vi "Canwrite_jetson_R.vi"(10 "Control param in":T1) -> (2 "배열":T2(array[cluster]))   [LabVIEW 2019]
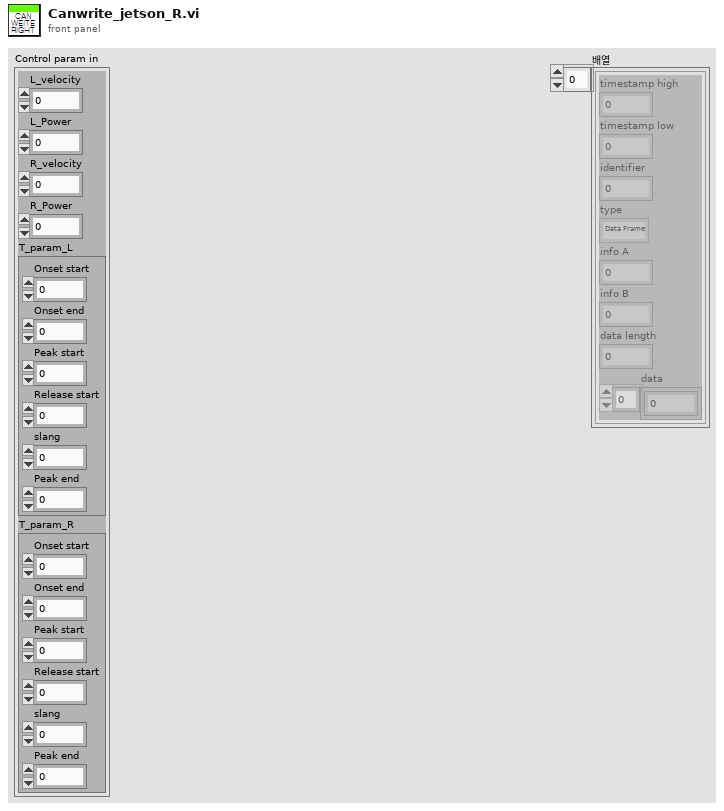
[diagram p1: front panel]
types:
  T1 = cluster{"L_velocity":u32, "L_Power":sgl, "R_velocity":u32, "R_Power":sgl, "T_param_L":cluster{"Onset start":sgl, "Onset end":sgl, "Peak start":sgl, "Release start":sgl, "slang":sgl, "Peak end":sgl}, "T_param_R":cluster{"Onset start":sgl, "Onset end":sgl, "Peak start":sgl, "Release start":sgl, "slang":sgl, "Peak end":sgl}}
  T2 = cluster{"timestamp high":u32, "timestamp low":u32, "identifier":u32, "type":enum8{"Data Frame", "Remote Frame", "(reserved)", "(reserved) ", "(reserved)  ", "(reserved)   ", "Bus Error", "Transceiver Fault"}, "info A":u8, "info B":u8, "data length":u8, "data":u8[]}[]
  T3 = enum8{"Data Frame", "Remote Frame", "(reserved)", "(reserved) ", "(reserved)  ", "(reserved)   ", "Bus Error", "Transceiver Fault"}
  T4 = cluster{"timestamp high":u32, "timestamp low":u32, "identifier":u32, "type":enum8{"Data Frame", "Remote Frame", "(reserved)", "(reserved) ", "(reserved)  ", "(reserved)   ", "Bus Error", "Transceiver Fault"}, "info A":u8, "info B":u8, "data length":u8, "data":u8[]}
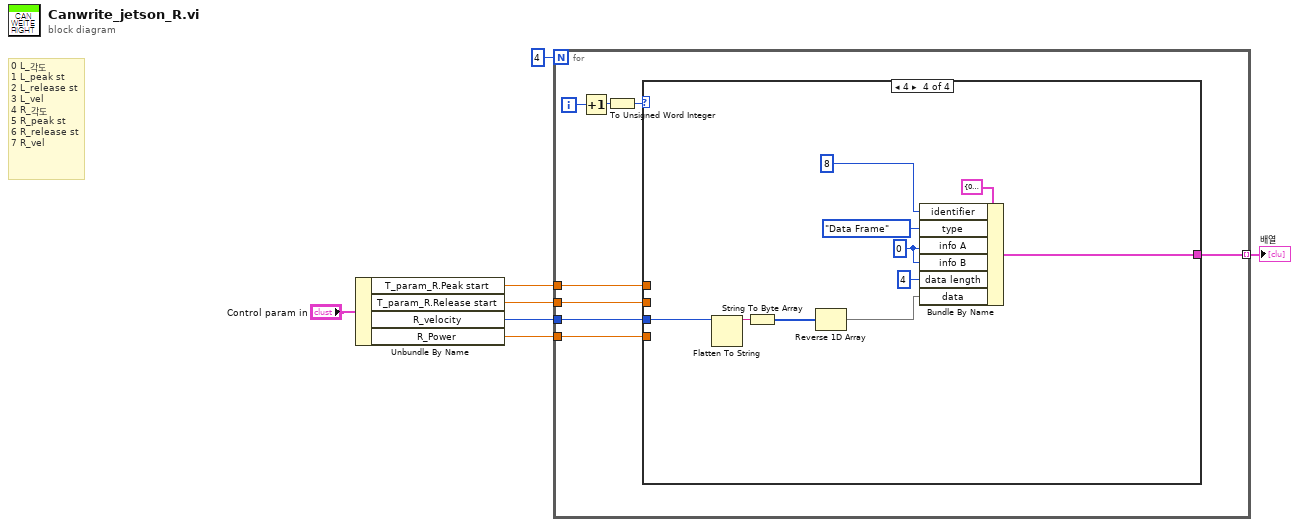
[diagram p0: block diagram]
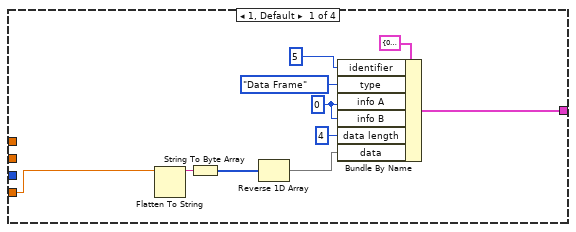
[diagram p2: hidden frame]
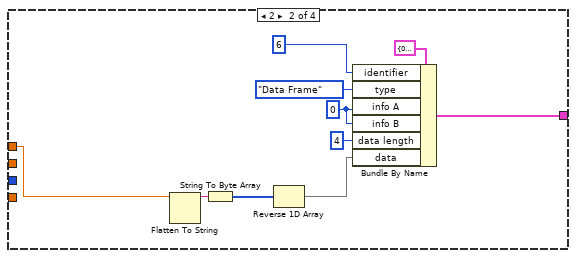
[diagram p3: hidden frame]
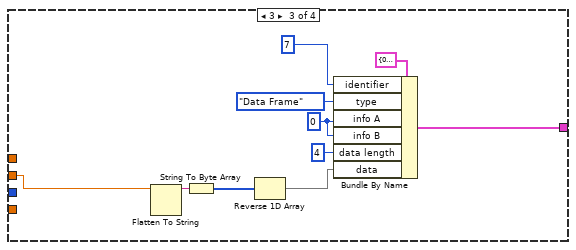
[diagram p4: hidden frame]
diagram:
  # "0 L_각도\n1 L_peak st\n2 L_release st\n3 L_vel\n4 R_각도\n5 R_peak st\n6 R_release st\n7 R_vel"
  n1 = Unbundle By Name("Control param in") -> ("T_param_R.Peak start"=w4:sgl, "T_param_R.Release start"=w3:sgl, "R_velocity"=w2:u32, "R_Power"=w1:sgl)
  n2 = for {
    N: 4 -> [_]
    tunnel: [w15] -> w6 mode=indexing
    tunnel: w4 -> [w11]
    tunnel: w3 -> [w10]
    tunnel: w2 -> [w9]
    tunnel: w1 -> [w8]
    i -> [w14]
    n3 = Increment(x=w14) -> (x+1=w13:i32)
    n4 = To Unsigned Word Integer(number=w13) -> (unsigned 16bit integer=w12:u16)
    n5 = case shown="4" w12 {
      tunnel: [w21 w31 w41 w51] -> w15
      tunnel: w11 -> [_ w27 _ _]
      tunnel: w10 -> [_ _ w37 _]
      tunnel: w9 -> [_ _ _ w47]
      tunnel: w8 -> [w17 _ _ _]
      frame 1, Default {
        w23 = u8 0 ("info A")
        n6 = Flatten To String(anything=w17) -> (data string=w20:string)  [unwired: 3 in, 2 out]
        n7 = String To Byte Array(string=w20) -> (unsigned byte array=w19:u8[])
        n8 = Reverse 1D Array(array=w19) -> (reversed array=w18:u8[])
        n9 = Bundle By Name(cluster=T4 {"timestamp high"=0, "timestamp low"=0, "identifier"=0, "type"=enum."Data Frame", "info A"=0, "info B"=0, "data length"=0, "data"=[0, 0, 0, 0, 0, 0, 0, 0]} ("출력 클러스터"), "identifier"=u32 5, "type"=T3."Data Frame", "info A"=w23, "info B"=w23, "data length"=u8 4, "data"=w18) -> (w21:T4)
      }
      frame 2 {
        w33 = u8 0 ("info A")
        n10 = Flatten To String(anything=w27) -> (data string=w30:string)  [unwired: 3 in, 2 out]
        n11 = String To Byte Array(string=w30) -> (unsigned byte array=w29:u8[])
        n12 = Reverse 1D Array(array=w29) -> (reversed array=w28:u8[])
        n13 = Bundle By Name(cluster=T4 {"timestamp high"=0, "timestamp low"=0, "identifier"=0, "type"=enum."Data Frame", "info A"=0, "info B"=0, "data length"=0, "data"=[0, 0, 0, 0, 0, 0, 0, 0]} ("출력 클러스터"), "identifier"=u32 6, "type"=T3."Data Frame", "info A"=w33, "info B"=w33, "data length"=u8 4, "data"=w28) -> (w31:T4)
      }
      frame 3 {
        w43 = u8 0 ("info A")
        n14 = Flatten To String(anything=w37) -> (data string=w40:string)  [unwired: 3 in, 2 out]
        n15 = String To Byte Array(string=w40) -> (unsigned byte array=w39:u8[])
        n16 = Reverse 1D Array(array=w39) -> (reversed array=w38:u8[])
        n17 = Bundle By Name(cluster=T4 {"timestamp high"=0, "timestamp low"=0, "identifier"=0, "type"=enum."Data Frame", "info A"=0, "info B"=0, "data length"=0, "data"=[0, 0, 0, 0, 0, 0, 0, 0]} ("출력 클러스터"), "identifier"=u32 7, "type"=T3."Data Frame", "info A"=w43, "info B"=w43, "data length"=u8 4, "data"=w38) -> (w41:T4)
      }
      frame 4 {
        w53 = u8 0 ("info A")
        n18 = Flatten To String(anything=w47) -> (data string=w50:string)  [unwired: 3 in, 2 out]
        n19 = String To Byte Array(string=w50) -> (unsigned byte array=w49:u8[])
        n20 = Reverse 1D Array(array=w49) -> (reversed array=w48:u8[])
        n21 = Bundle By Name(cluster=T4 {"timestamp high"=0, "timestamp low"=0, "identifier"=0, "type"=enum."Data Frame", "info A"=0, "info B"=0, "data length"=0, "data"=[0, 0, 0, 0, 0, 0, 0, 0]} ("출력 클러스터"), "identifier"=u32 8, "type"=T3."Data Frame", "info A"=w53, "info B"=w53, "data length"=u8 4, "data"=w48) -> (w51:T4)
      }
    }
  }
  "배열" <- w6
